vi "Select_Sheet.vi"(6 "Worksheet Number":i32, 8 "error in (no error)":errorcluster, 11 "Automation Refnum in":refnum<k7>) -> (0 "error out":errorcluster, 3 "Automation Refnum out":refnum<k7>, 5 "Sheets Refnum":refnum<k7>)   [LabVIEW 2014]
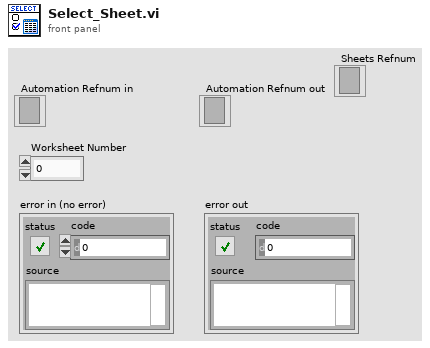
[diagram p1: front panel]
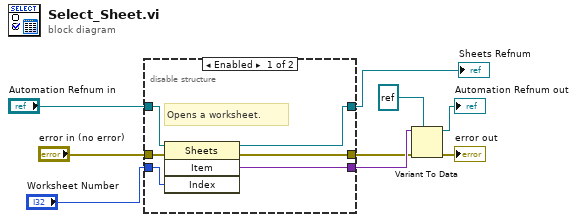
[diagram p0: block diagram]
diagram:
  n1 = disable-structure shown="Enabled" {
    disable-tunnel: [w15 w17] -> w1
    disable-tunnel: [w14 w18] -> w2
    disable-tunnel: [w13 w16] -> w4
    disable-tunnel: "error in (no error)" -> [w12 w17]
    disable-tunnel: "Automation Refnum in" -> [w11 w18]
    disable-tunnel: "Worksheet Number" -> [w10 w16]
    frame Enabled {
      # "Opens a worksheet."
      n2 = invoke class="Sheets" method="Item"(reference=w11, error in=w12, "Index"=w10) -> (reference out=w14:refnum<k7>, error out=w15:errorcluster, "Item"=w13:variant)  [unwired: 1 in, 1 out]
    }
    frame Disabled {
    }
  }
  "Sheets Refnum" <- w2
  n3 = Variant To Data(error in=w1, type=refnum<k7> refnum ("Excel._Worksheet"), Variant=w4) -> (data=→"Automation Refnum out":refnum<k7>, error out=→"error out":errorcluster)
